vi "Customer Identifier.vi"(0 "VISA resource name":refnum<visa-resource-name>, 1 "Unit Address (1)":u8=1 min=1 max=254, 5 "Customer Identifier":u16 max=9999, 11 "error in (no error)":errorcluster) -> (4 "VISA resource name out":refnum<visa-resource-name>, 15 "error out":errorcluster)   [LabVIEW 2010, in "Eurotherm 32xx Series.lvlib"]
doc: "This VI sets Customer Identifier.\n\nA customer Identifier is provided to allow a number to be stored in the instrument.\n\nThis number has no use in the instruments application, it is provided as a method of identifying the instrument to the customer only."
uses:
  <instrlib>/Eurotherm 32xx Series/Eurotherm 32xx Series.lvlib
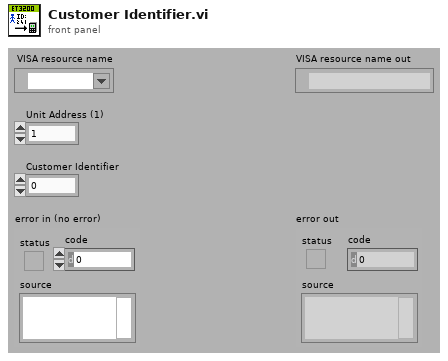
[diagram p1: front panel]
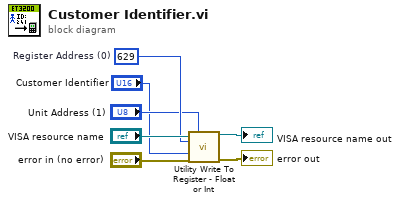
[diagram p0: block diagram]
diagram:
  w5 = u16 629  # Register Address (0)
  n1 = call <instrlib>:"Utility Write To Register - Float or Int.vi"("VISA resource name"="VISA resource name", "Unit Address (1)"="Unit Address (1)", "Register Address (0)"=w5, "Data (0)"="Customer Identifier", "error in (no error)"="error in (no error)") -> ("VISA resource name out"=→"VISA resource name out":refnum<visa-resource-name>, "error out"=→"error out":errorcluster)  [unwired: 9 in]
